vi "Create Sequence View.vi"(8 "error in (no error)":errorcluster, 10 "Subpanel":refnum<vi>, 11 "TSnax UI Manager in":refnum<class "TSnax UI Manager.lvclass">) -> (0 "error out":errorcluster, 2 "Sequence View":refnum<class "SequenceViewPanel.lvclass">, 3 "TSnax UI Manager out":refnum<class "TSnax UI Manager.lvclass">)   [LabVIEW 2020, in "TSnax UI.lvlib" / "TSnax UI Manager.lvclass"]
uses:
  TSnax UI Manager.lvclass
  TSnax UI Manager.lvclass/TSnax UI Manager.ctl
  <vilib>/IlluminatedG/IG OOPanel/OOPanel/Manager/Manager.lvclass
  SequenceViewPanel/SequenceViewPanel.lvclass
  C:/Program Files (x86)/National Instruments/LabVIEW 2020/vi.lib/IlluminatedG/IG OOPanel/OOPanel/Panel/Panel.lvclass
  C:/dev/illuminated-g/tsnax/TSnax UI/SequenceViewPanel/SequenceViewPanel.lvclass
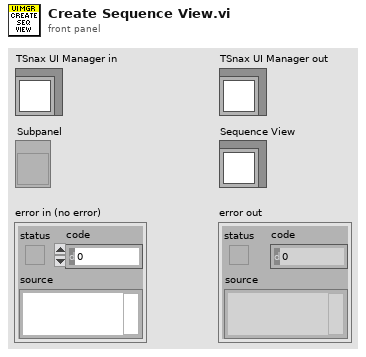
[diagram p1: front panel]
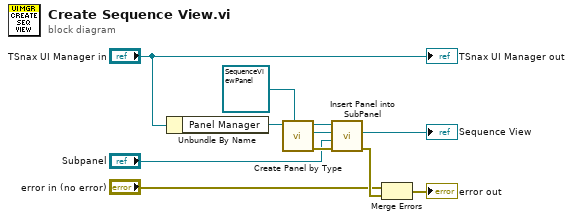
[diagram p0: block diagram]
diagram:
  n1 = Unbundle By Name("TSnax UI Manager in") -> ("Panel Manager"=w11:refnum<class "Manager.lvclass">)
  n2 = call <vilib>:"Create Panel by Type.vi"("Panel Type"=refnum<class "SequenceViewPanel.lvclass"> refnum ("Sequence View"), "Manager in"=w11) -> ("error out"=w8:errorcluster, "Panel"=w9:refnum<class "SequenceViewPanel.lvclass">, "Manager out"=w10:refnum<class "Manager.lvclass">)  [unwired: 7 in]
  n3 = call <vilib>:"Insert Panel into SubPanel.vi"("error in (no error)"=w8, "SubPanel"="Subpanel", "Panel In"=w9, "Manager in"=w10) -> ("error out"=w7:errorcluster, "Panel"=→"Sequence View":refnum<class "SequenceViewPanel.lvclass">)  [unwired: 5 in, 1 out]
  n4 = Merge Errors("error in (no error)", w7) -> (→"error out":errorcluster)
  "TSnax UI Manager out" <- "TSnax UI Manager in"
